vi "Box.vi"(10 "data":i32) -> (2 "CustomeData out":refnum<class "CustomeData.lvclass">)   [LabVIEW 2021, in "CustomeData.lvclass"]
uses:
  CustomeData.lvclass
  CustomeData.lvclass/CustomeData.ctl
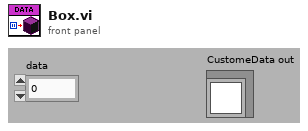
[diagram p1: front panel]
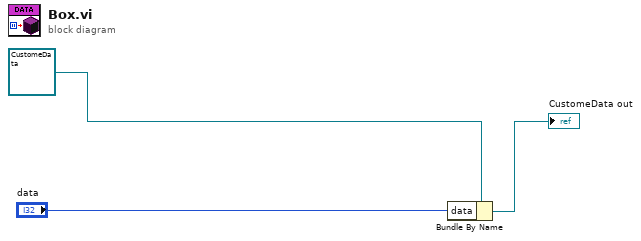
[diagram p0: block diagram]
diagram:
  n1 = Bundle By Name(cluster=refnum<class "CustomeData.lvclass"> refnum ("CustomeData in"), "data"="data") -> (→"CustomeData out":refnum<class "CustomeData.lvclass">)
